vi "JoystickControls.vi"() -> (3 "output cluster":T1)   [LabVIEW 2016]
uses:
  Controls.ctl
  References/Refnums.vi
  <vilib>/Rock Robotics/WPI/Utilities/WPI_GetSetVariantRefNum.vi
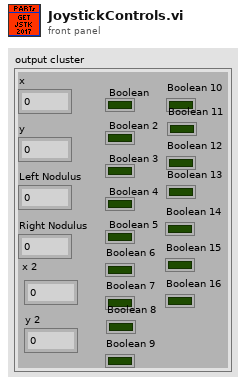
[diagram p1: front panel]
types:
  T1 = typedef "Controls.ctl" = cluster{"x":dbl, "y":dbl, "Left Nodulus":dbl, "Right Nodulus":dbl, "Boolean":bool, "Boolean 2":bool, "Boolean 3":bool, "Boolean 4":bool, "Boolean 5":bool, "Boolean 6":bool, "Boolean 7":bool, "Boolean 8":bool, "Boolean 9":bool, "Boolean 10":bool, "Boolean 11":bool, "Boolean 12":bool, "Boolean 13":bool, "Boolean 14":bool, "Boolean 15":bool, "x 2":dbl, "y 2":dbl, "Boolean 16":bool}
  T2 = typedef "WPI_JoystickDevRef.ctl" = cluster{"Device":T3}
  T3 = typedef "WPI_JoystickDeviceEnum.ctl" = enum16{"USB 0", "USB 1", "USB 2", "USB 3", "USB 4", "USB 5"}
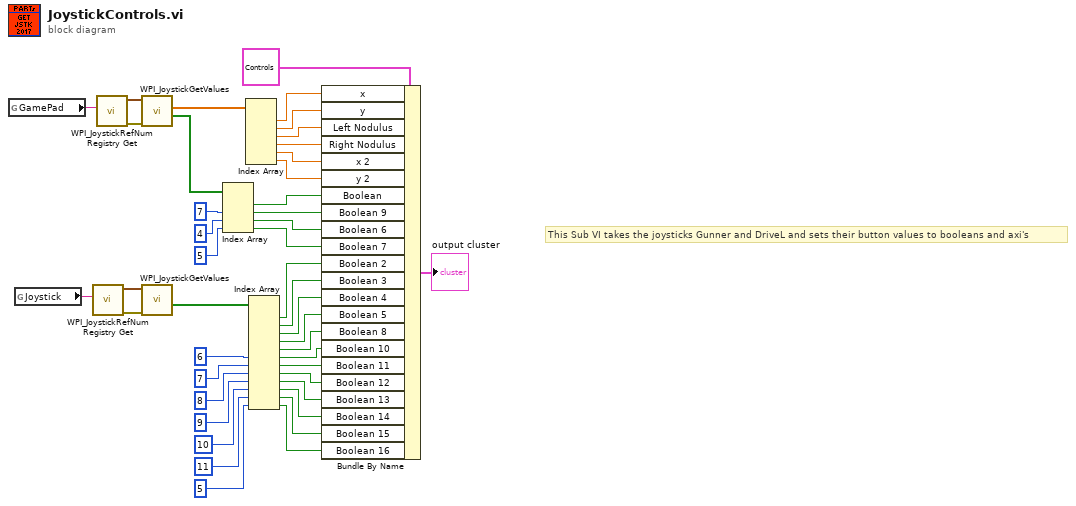
[diagram p0: block diagram]
diagram:
  # "This Sub VI takes the joysticks Gunner and DriveL and sets their button values to booleans and axi's"
  n1 = global read "Refnums.vi" "GamePad"() -> (w2:string)
  n2 = global read "Refnums.vi" "Joystick"() -> (w1:string)
  n3 = call <vilib>:"WPI_JoystickRefNum Registry Get.vi"("refnum name"=w1) -> ("error out"=w5:errorcluster, "JoystickDevRef"=w4:T2)  [unwired: 9 in]
  n4 = call <vilib>:"WPI_JoystickRefNum Registry Get.vi"("refnum name"=w2) -> ("error out"=w9:errorcluster, "JoystickDevRef"=w8:T2)  [unwired: 9 in]
  n5 = call <vilib>:"WPI_JoystickGetValues.vi"("error in (no error)"=w9, "JoystickDevRef"=w8) -> ("Buttons"=w6:bool[], "Axes"=w7:dbl[])  [unwired: 5 in, 3 out]
  n6 = call <vilib>:"WPI_JoystickGetValues.vi"("error in (no error)"=w5, "JoystickDevRef"=w4) -> ("Buttons"=w3:bool[])  [unwired: 5 in, 4 out]
  n7 = Index Array(array=w6, index #2=7 ("index"), index #3=4 ("index"), index #4=5 ("index")) -> (element #1=w41:bool, element #2=w39:bool, element #3=w36:bool, element #4=w35:bool)  [unwired: 1 in]
  n8 = Index Array(array=w7) -> (element #1=w12:dbl, element #2=w13:dbl, element #3=w14:dbl, element #4=w15:dbl, element #5=w16:dbl, element #6=w17:dbl)  [unwired: 6 in]
  n9 = Index Array(array=w3, index #6=6 ("index"), index #7=7 ("index"), index #8=8 ("index"), index #9=9 ("index"), index #10=10 ("index"), index #11=11 ("index"), index #12=5 ("index")) -> (element #1=w34:bool, element #2=w33:bool, element #3=w32:bool, element #4=w31:bool, element #5=w30:bool, element #6=w28:bool, element #7=w26:bool, element #8=w24:bool, element #9=w22:bool, element #10=w20:bool, element #11=w18:bool, element #12=w10:bool)  [unwired: 5 in]
  n10 = Bundle By Name(cluster=T1 {"x"=0.0, "y"=0.0, "Left Nodulus"=0.0, "Right Nodulus"=0.0, "Boolean"=FALSE, "Boolean 2"=FALSE, "Boolean 3"=FALSE, "Boolean 4"=FALSE, "Boolean 5"=FALSE, "Boolean 6"=FALSE, "Boolean 7"=FALSE, "Boolean 8"=FALSE, "Boolean 9"=FALSE, "Boolean 10"=FALSE, "Boolean 11"=FALSE, "Boolean 12"=FALSE, "Boolean 13"=FALSE, "Boolean 14"=FALSE, "Boolean 15"=FALSE, "x 2"=0.0, "y 2"=0.0, "Boolean 16"=FALSE} ("input cluster"), "x"=w12, "y"=w13, "Left Nodulus"=w14, "Right Nodulus"=w15, "x 2"=w16, "y 2"=w17, "Boolean"=w41, "Boolean 9"=w39, "Boolean 6"=w36, "Boolean 7"=w35, "Boolean 2"=w34, "Boolean 3"=w33, "Boolean 4"=w32, "Boolean 5"=w31, "Boolean 8"=w30, "Boolean 10"=w28, "Boolean 11"=w26, "Boolean 12"=w24, "Boolean 13"=w22, "Boolean 14"=w20, "Boolean 15"=w18, "Boolean 16"=w10) -> (→"output cluster":T1)
